vi "TurretAngleControl.vi"(0 "TurretMotorControlDevRef":T1={"DeviceStatus"={"status"=FALSE, "code"=0, "source"=""}, "Type"=enum."PWM", "PWM"={"PWM Channel"=enum."PWM 1", "DeadBand"={"Name"="", "maxPositivePwm"=0, "minPositivePwm"=0, "centerPwm"=0, "maxNegativePwm"=0, "minNegativePwm"=0, "angularRange"=0}}, "CAN"={"Device Number"=0, "SetOutput VI Ref"=variant(enum8{"Percent VBus", "Current", "Speed", "Position", "Voltage"} enum."Percent VBus"), "GetOutput VI Ref"=variant(refnum<k1> refnum), "Enable VI Ref"=variant(dbl 12.0), "Disable VI Ref"=variant(enum8{"Percent VBus", "Speed", "Position", "Slave", "Unchanged / Invalid", "Voltage Compensation", "Current", "Motion Profile"} enum."Percent VBus"), "Data"=variant}, "Invert"=FALSE, "DIO PWM"={"PWM \"Enable\" Channel"=enum."Invalid", "DIOChannel"=enum."Invalid", "PWM Rate"=0.0}}, 1 "Activate Auto":bool, 2 "MaxDegrees":dbl, 5 "Homing":bool, 7 "MinDegrees":dbl, 9 "MotorConfig":T6={"CAN Address"=0, "Invert"=FALSE, "InvertSensor"=FALSE, "Unit Conversion Factor"=0.0, "Brake Mode"=enum."Override to Brake", "Reverse Limt Switch Mode"=enum."Disabled", "Forward Limt Swith Mode"=enum."Disabled", "PWM Channel"=enum."Invalid", "Motor Controller Type"=enum."Talon SRX", "Peak Current (A)"=0, "Continuous Current (A)"=0, "Peak Duration (ms)"=0, "Current Limit Enable"=FALSE}, 11 "SetPoint(Deg)":dbl, 12 "ManualControl":dbl min=0.0 max=1.0) -> (6 "Manual?":bool, 15 "Current Position (Deg)":dbl)   [LabVIEW 2019]
uses:
  ArgosLib/Config/ConfigComponents/TypeDefs/Config_PIDParams.ctl
  ArgosLib/Config/ConfigComponents/TypeDefs/Config_Motor.ctl
  <vilib>/Rock Robotics/WPI/ThirdParty/Phoenix-LabVIEW/Motor Controller/Controls/CTRE_Phoenix_MotorControl_NeutralMode.ctl
  <vilib>/Rock Robotics/WPI/ThirdParty/Phoenix-LabVIEW/Motor Controller/Controls/CTRE_Phoenix_MotorControl_LimitSwitchNormal.ctl
  <vilib>/Rock Robotics/SystemInterfaces/DIO/FPGA_DIOPWMChannel.ctl
  ArgosLib/Config/ConfigComponents/TypeDefs/Config_MotorCtrlType.ctl
  <vilib>/Rock Robotics/WPI/MotorControl/WPI_MotorControlDeviceRef.ctl
  <vilib>/Rock Robotics/WPI/MotorControl/WPI_MotorControlType.ctl
  <vilib>/Rock Robotics/WPI/PWM/WPI_PWMDeadband.ctl
  <vilib>/Rock Robotics/SystemInterfaces/DIO/FPGA_DIOChannel.ctl
  ArgosLib/Signal Processing/TypeDefs/EdgeDetector_Type.ctl
  <vilib>/Rock Robotics/WPI/ThirdParty/Phoenix-LabVIEW/Motor Controller/Controls/CTRE_Phoenix_MotorControl_ControlMode.ctl
  <vilib>/Rock Robotics/WPI/ThirdParty/Phoenix-LabVIEW/Motor Controller/Get/CTRE_Phoenix_MotorController_GetSelectedSensorData.vi
  ArgosLib/ArgosLib.lvlib
panel:
  out "Waveform Chart":cluster{dbl, "SetPoint(Deg)":dbl}(graph)
  in  "PIDParams":T10
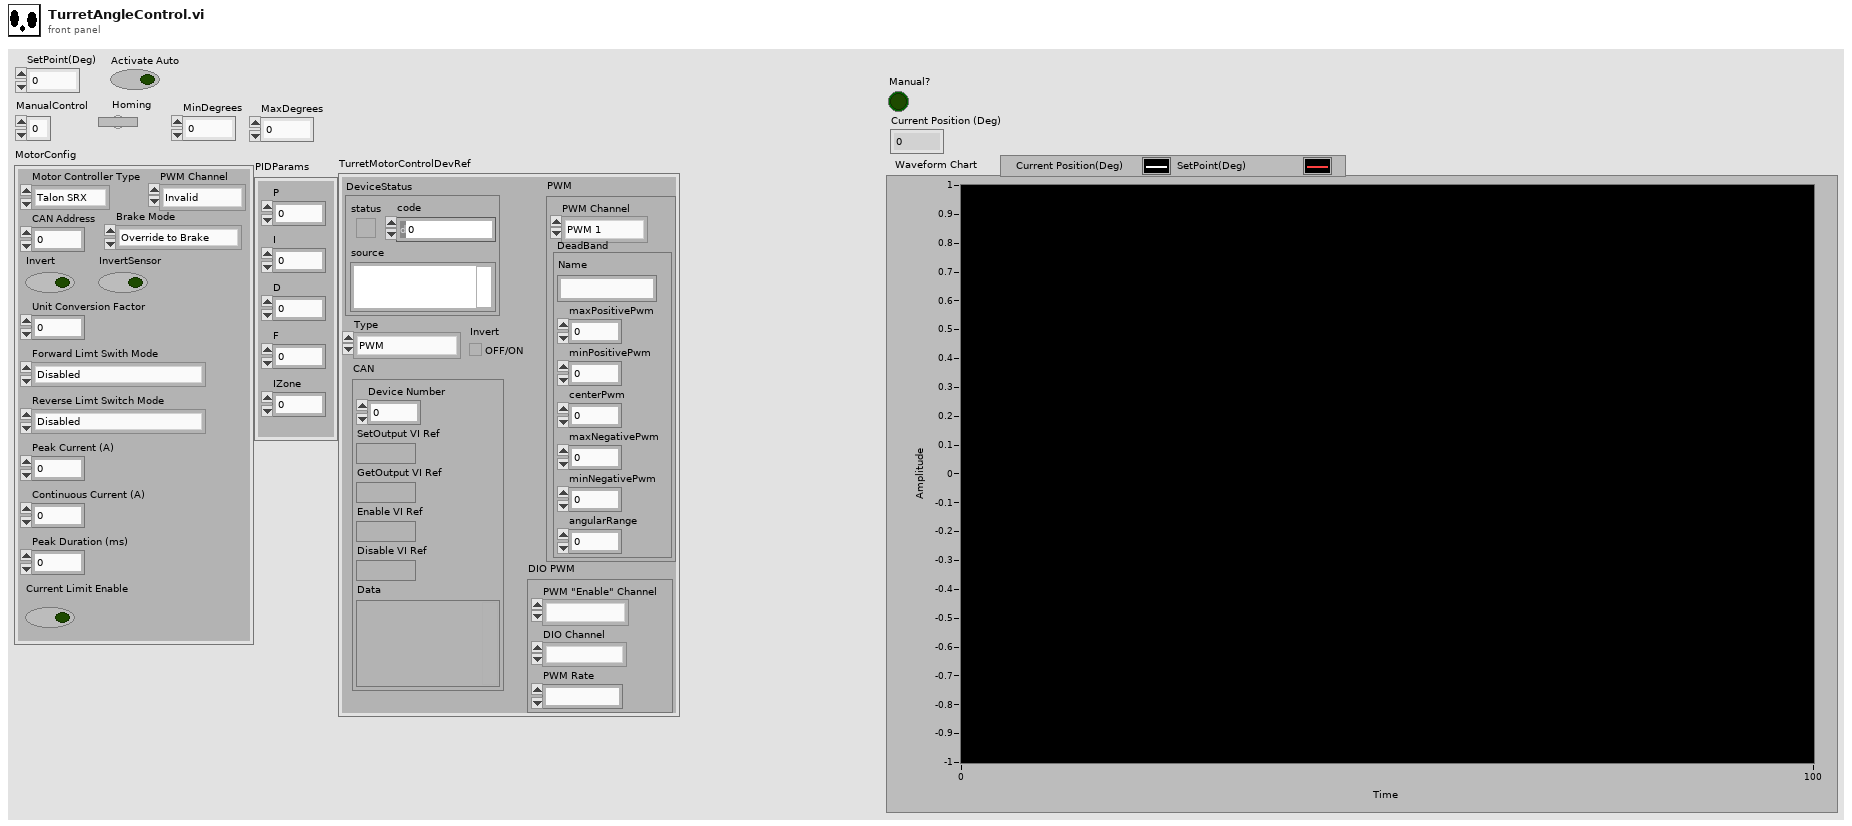
[diagram p1: front panel]
types:
  T1 = typedef "WPI_MotorControlDeviceRef.ctl" = cluster{"DeviceStatus":errorcluster, "Type":T2, "PWM":cluster{"PWM Channel":T3, "DeadBand":T4}, "CAN":cluster{"Device Number":u8, "SetOutput VI Ref":variant, "GetOutput VI Ref":variant, "Enable VI Ref":variant, "Disable VI Ref":variant, "Data":variant}, "Invert":bool, "DIO PWM":cluster{"PWM \"Enable\" Channel":T3, "DIOChannel":T5, "PWM Rate":dbl}}
  T2 = typedef "WPI_MotorControlType.ctl" = enum16{"PWM", "CAN", "DIO PWM"}
  T3 = typedef "FPGA_DIOPWMChannel.ctl" = enum8{"PWM 0", "PWM 1", "PWM 2", "PWM 3", "PWM 4", "PWM 5", "PWM 6", "PWM 7", "PWM 8", "PWM 9", "PWM MXP 0", "PWM MXP 1", "PWM MXP 2", "PWM MXP 3", "PWM MXP 4", "PWM MXP 5", "PWM MXP 6", "PWM MXP 7", "PWM MXP 8", "PWM MXP 9", "Invalid"}
  T4 = typedef "WPI_PWMDeadband.ctl" = cluster{"Name":string, "maxPositivePwm":i32, "minPositivePwm":i32, "centerPwm":i32, "maxNegativePwm":i32, "minNegativePwm":i32, "angularRange":u16}
  T5 = typedef "FPGA_DIOChannel.ctl" = enum8{"DIO 0", "DIO 1", "DIO 2", "DIO 3", "DIO 4", "DIO 5", "DIO 6", "DIO 7", "DIO 8", "DIO 9", "DIO MXP 0", "DIO MXP 1", "DIO MXP 2", "DIO MXP 3", "DIO MXP 4", "DIO MXP 5", "DIO MXP 6", "DIO MXP 7", "DIO MXP 8", "DIO MXP 9", "DIO MXP 10", "DIO MXP 11", "DIO MXP 12", "DIO MXP 13", "DIO MXP 14", "DIO MXP 15", "SPI Port CS1", "SPI Port CS2", "SPI Port CS3", "SPI Port MISO", "SPI Port MOSI", "Invalid"}
  T6 = typedef "ArgosLib.lvlib/Config_Motor.ctl" = cluster{"CAN Address":u8, "Invert":bool, "InvertSensor":bool, "Unit Conversion Factor":dbl, "Brake Mode":T7, "Reverse Limt Switch Mode":T8, "Forward Limt Swith Mode":T8, "PWM Channel":T3, "Motor Controller Type":T9, "Peak Current (A)":i32, "Continuous Current (A)":i32, "Peak Duration (ms)":i32, "Current Limit Enable":bool}
  T7 = typedef "CTRE_Phoenix_MotorControl_NeutralMode.ctl" = enum8{"EEPROMSetting", "Override to Coast", "Override to Brake"}
  T8 = typedef "CTRE_Phoenix_MotorControl_LimitSwitchNormal.ctl" = enum16{"Normally Open", "Normally Closed", "Disabled"}
  T9 = typedef "ArgosLib.lvlib/Config_MotorCtrlType.ctl" = enum16{"Disabled", "Talon SRX", "Talon SR", "Venom", "Spark MAX"}
  T10 = typedef "ArgosLib.lvlib/Config_PIDParams.ctl" = cluster{"P":dbl, "I":dbl, "D":dbl, "F":dbl, "IZone":dbl}
  T11 = typedef "ArgosLib.lvlib/EdgeDetector_Type.ctl" = enum16{"RisingEdge", "FallingEdge", "Both"}
  T12 = cluster{"P":bool, "I":bool, "D":bool, "F":bool, "IZone":bool}
  T13 = typedef "CTRE_Phoenix_MotorControl_ControlMode.ctl" = u16
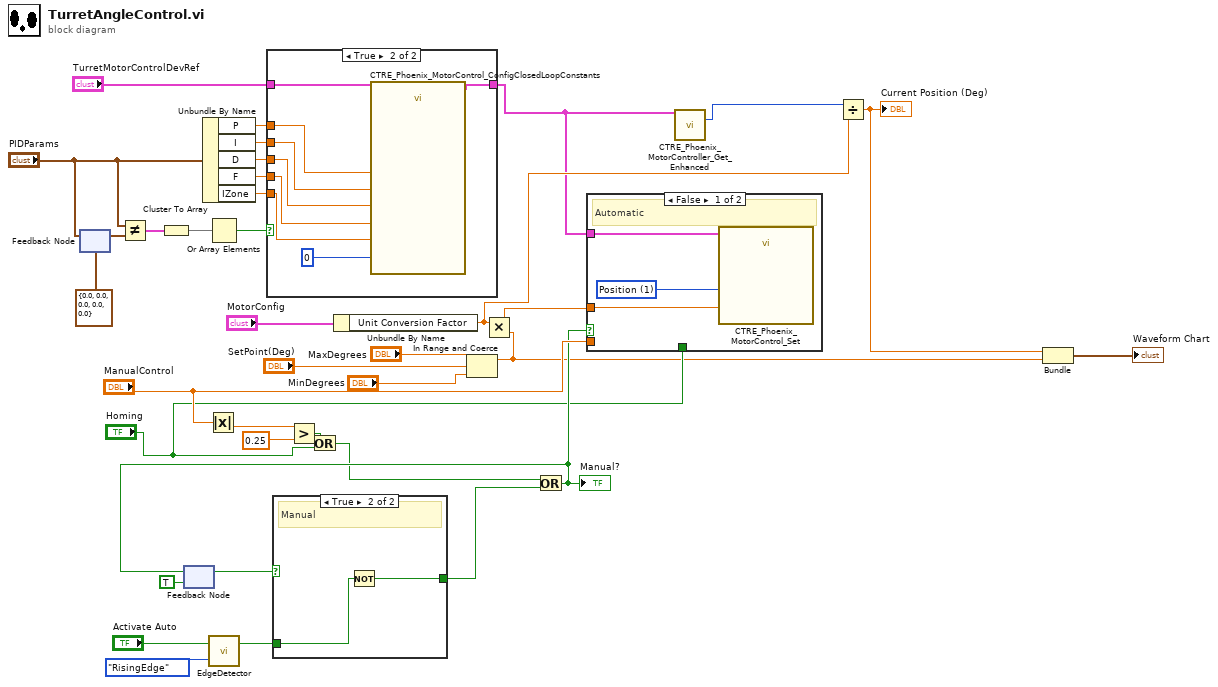
[diagram p0: block diagram]
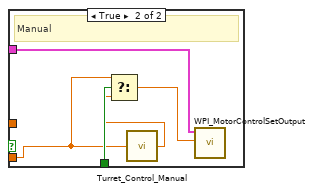
[diagram p3: hidden frame]
diagram:
  n1 = feedback-in #1("PIDParams") -> ()
  n2 = feedback #1(T10 {"P"=0.0, "I"=0.0, "D"=0.0, "F"=0.0, "IZone"=0.0} ("PIDParams")) -> (w35:T10)
  n3 = Not Equal?(x="PIDParams", y=w35) -> (x != y?=w34:T12)
  n4 = Cluster To Array(cluster=w34) -> (array=w33:bool[])
  n5 = feedback #2(TRUE) -> (w20:bool)
  n6 = Unbundle By Name("PIDParams") -> ("P"=w29:dbl, "I"=w28:dbl, "D"=w27:dbl, "F"=w26:dbl, "IZone"=w25:dbl)
  n7 = Absolute Value(x="ManualControl") -> (abs(x)=w21:dbl)
  n8 = Or Array Elements(Boolean array=w33) -> (logical OR=w31:bool)
  n9 = call "EdgeDetector.vi"("DetectorType"=EdgeDetector_Type."RisingEdge", "Input"="Activate Auto") -> ("Edge"=w2:bool)
  n10 = case shown="True" w31 {
    tunnel: "TurretMotorControlDevRef" -> [w37 w45]
    tunnel: w29 -> [_ w42]
    tunnel: w28 -> [_ w41]
    tunnel: w27 -> [_ w40]
    tunnel: w26 -> [_ w39]
    tunnel: w25 -> [_ w38]
    tunnel: [w37 w44] -> w12
    frame False {
    }
    frame True {
      n11 = call <vilib>:"CTRE_Phoenix_MotorControl_ConfigClosedLoopConstants.vi"("PhoenixMotorControlDevRef"=w45, "slotIdx"=0, "P"=w42, "I"=w41, "D"=w40, "F"=w39, "I Zone"=w38) -> ("PhoenixMotorControlDevRef"=w44:T1)  [unwired: 7 in, 1 out]
    }
  }
  n12 = case shown="True" w20 {
    selector: w20 -> [w46 _]
    tunnel: [w46 w48] -> w19
    tunnel: w2 -> [_ w47]
    frame False {
      # "Automatic"
    }
    frame True {
      # "Manual"
      n13 = Not(x=w47) -> (.not. x?=w48:bool)
    }
  }
  n14 = Greater?(x=w21, y=0.25) -> (0:w18:bool)
  n15 = Or(x=w18, y="Homing") -> (x .or. y?=w9:bool)
  n16 = Unbundle By Name("MotorConfig") -> ("Unit Conversion Factor"=w13:dbl)
  n17 = In Range and Coerce(upper limit="MaxDegrees", x="SetPoint(Deg)", lower limit="MinDegrees") -> (coerced(x)=w4:dbl)  [unwired: 1 out]
  n18 = Multiply(x=w13, y=w4) -> (x*y=w23:dbl)
  n19 = Or(x=w9, y=w19) -> (x .or. y?=w16:bool)
  "Manual?" <- w16
  n20 = feedback-in #2(w16) -> ()
  n21 = case shown="False" w16 {
    tunnel: w23 -> [w51 _]
    tunnel: "ManualControl" -> [_ w53]
    tunnel: w12 -> [w49 w56]
    tunnel: "Homing" -> [_ w55]
    frame False {
      w50 = T13 1 items=["PercentOutput"=0, "Position"=1, "Velocity"=2, "Current"=3, "Follower"=5, "MotionProfile"=6, "MotionMagic"=7, "MotionProfileArc"=10, "Disabled"=15] ("Control Mode")
      # "Automatic"
      n22 = call <vilib>:"CTRE_Phoenix_MotorControl_Set.vi"("Output"=w51, "Control Mode"=w50, "PhoenixMotorControlDevRef"=w49) -> ()  [unwired: 7 in, 2 out]
    }
    frame True {
      # "Manual"
      n23 = call "Turret_Control_Manual.vi"("Rotate_Command"=w53) -> ("TurretMotorCommand"=w52:dbl)
      n24 = Select(t=w53, s=w55, f=w52) -> (s? t:f=w54:dbl)
      n25 = call <vilib>:"WPI_MotorControlSetOutput.vi"("Output"=w54, "MotorControlDevRef"=w56) -> ()  [unwired: 7 in, 3 out]
    }
  }
  n26 = call-poly <vilib>:"CTRE_Phoenix_MotorController_Get_Enhanced.vi"("PhoenixMotorControlDevRef"=w12) -> ("Position (Raw Sensor Units)"=w14:i32)  [unwired: 11 in, 3 out]
  n27 = Divide(x=w14, y=w13) -> (x/y=w11:dbl)
  "Current Position (Deg)" <- w11
  n28 = Bundle(w11, "MaxDegrees"=w4) -> (→"Waveform Chart":cluster{dbl, "MaxDegrees":dbl})  [unwired: 1 in]
